vi "updateCamera.vi"(8 "error in (no error)":errorcluster, 10 "data":T1, 11 "AtomChipHWC in":refnum<class "AtomChipHWC.lvclass">) -> (0 "error out":errorcluster, 3 "AtomChipHWC out":refnum<class "AtomChipHWC.lvclass">)   [LabVIEW 2011, in "Hardware.lvlib" / "HWControllers.lvlib" / "AtomChipHWC.lvclass"]
uses:
  AtomChipHWC.lvclass
  AtomChipHWC.lvclass/AtomChipHWC.ctl
  Network Controllers/NetworkCamera/NetworkCamera.lvclass
panel:
  # "start - stop in type?"
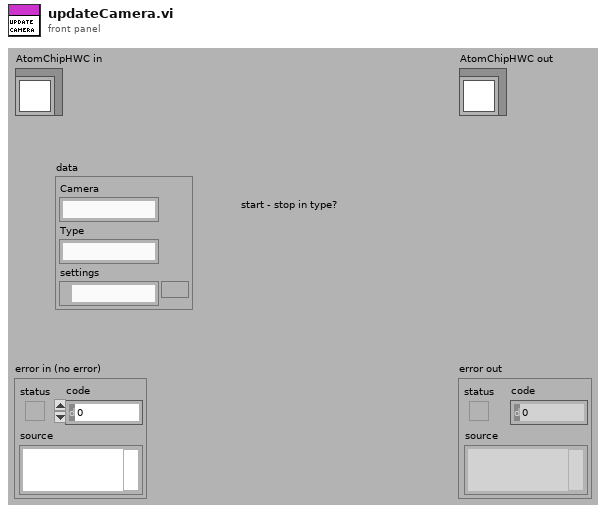
[diagram p1: front panel]
types:
  T1 = cluster{"Camera":string, "Type":string, "settings":path}
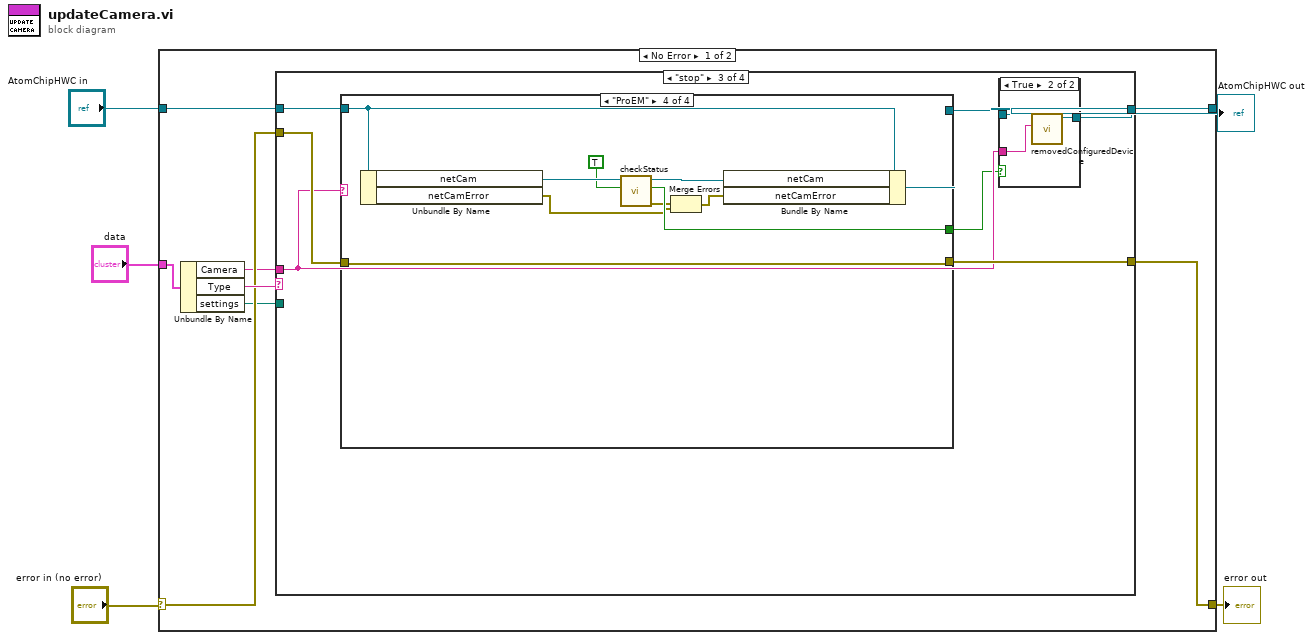
[diagram p0: block diagram]
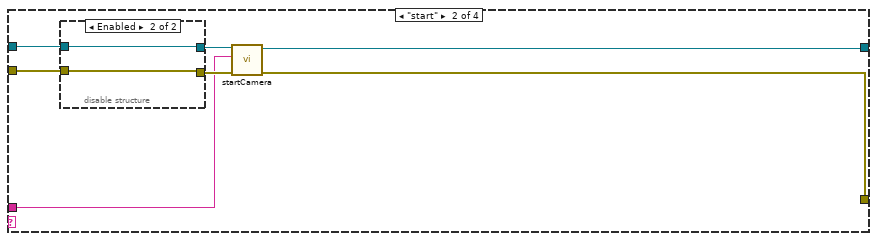
[diagram p3: hidden frame]
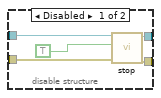
[diagram p4: hidden frame]
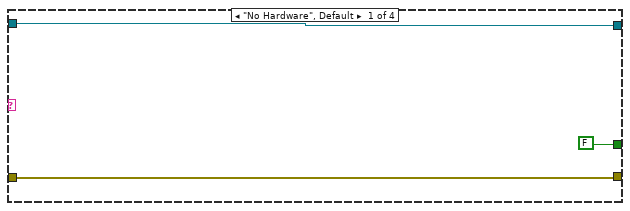
[diagram p6: hidden frame]
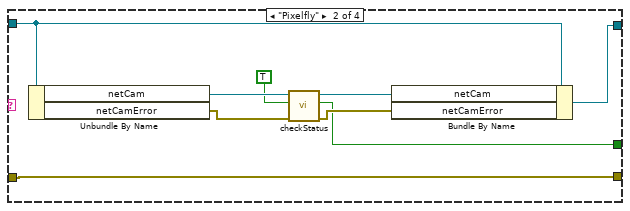
[diagram p7: hidden frame]
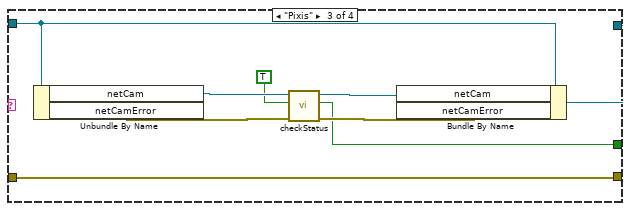
[diagram p8: hidden frame]
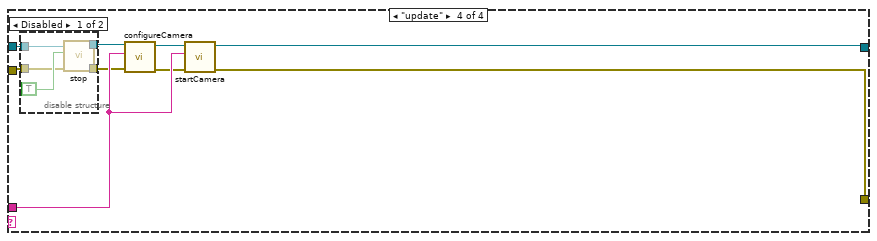
[diagram p9: hidden frame]
diagram:
  n1 = case shown="No Error" "error in (no error)" {
    selector: "error in (no error)" -> [w10 w88]
    tunnel: [w9 w89] -> w4
    tunnel: "AtomChipHWC in" -> [w11 w89]
    tunnel: [w8 w88] -> w2
    tunnel: "data" -> [w13 _]
    frame No Error {
      n2 = Unbundle By Name(w13) -> ("Camera"=w6:string, "Type"=w12:string, "settings"=w7:path)
      n3 = case shown="\"stop\"" w12 {
        tunnel: w11 -> [w15 w22 w36 w75]
        tunnel: w10 -> [w14 w21 w35 w72]
        tunnel: [w15 w18 w32 w77] -> w9
        tunnel: [w14 w17 w34 w76] -> w8
        tunnel: w7 -> [_ _ _ _]
        tunnel: w6 -> [_ w16 w31 w79]
        frame "", Default {
        }
        frame "start" {
          n4 = disable-structure shown="Enabled" {
            disable-tunnel: w22 -> [w26 w29]
            disable-tunnel: w21 -> [w25 w28]
            disable-tunnel: [w24 w29] -> w20
            disable-tunnel: [w23 w28] -> w19
            frame Disabled {
              n5 = call-dynamic "stop.vi"("error in (no error)"=w25, "stop?"=TRUE, "AtomChipHWC in"=w26) -> ("error out"=w23:errorcluster, "AtomChipHWC out"=w24:refnum<class "AtomChipHWC.lvclass">)  [unwired: 6 in, 1 out]
            }
            frame Enabled {
            }
          }
          n6 = call "startCamera.vi"("error in (no error)"=w19, "camera"=w16, "AtomChipHWC in"=w20) -> ("error out"=w17:errorcluster, "AtomChipHWC out"=w18:refnum<class "AtomChipHWC.lvclass">)  [unwired: 7 in]
        }
        frame "stop" {
          n7 = case shown="\"ProEM\"" w31 {
            tunnel: [w43 w51 w60 w70] -> w33
            tunnel: [w41 w44 w53 w65] -> w34
            tunnel: w36 -> [w43 w52 w61 w71]
            tunnel: [FALSE w45 w54 w66] -> w30
            tunnel: w35 -> [w41 w44 w53 w65]
            frame "No Hardware", Default {
            }
            frame "Pixelfly" {
              n8 = Unbundle By Name(w52) -> ("netCam"=w49:refnum<class "NetworkCamera.lvclass">, "netCamError"=w48:errorcluster)
              n9 = call-dynamic "checkStatus.vi"("error in (no error)"=w48, "stop"=TRUE, "NetworkCamera in"=w49) -> ("error out"=w47:errorcluster, "stopped?"=w45:bool, "NetworkCamera out"=w50:refnum<class "NetworkCamera.lvclass">)  [unwired: 6 in]
              n10 = Bundle By Name(cluster=w52, "netCam"=w50, "netCamError"=w47) -> (w51:refnum<class "AtomChipHWC.lvclass">)
            }
            frame "Pixis" {
              n11 = Unbundle By Name(w61) -> ("netCam"=w58:refnum<class "NetworkCamera.lvclass">, "netCamError"=w57:errorcluster)
              n12 = call-dynamic "checkStatus.vi"("error in (no error)"=w57, "stop"=TRUE, "NetworkCamera in"=w58) -> ("error out"=w56:errorcluster, "stopped?"=w54:bool, "NetworkCamera out"=w59:refnum<class "NetworkCamera.lvclass">)  [unwired: 6 in]
              n13 = Bundle By Name(cluster=w61, "netCam"=w59, "netCamError"=w56) -> (w60:refnum<class "AtomChipHWC.lvclass">)
            }
            frame "ProEM" {
              n14 = Unbundle By Name(w71) -> ("netCam"=w68:refnum<class "NetworkCamera.lvclass">, "netCamError"=w63:errorcluster)
              n15 = call-dynamic "checkStatus.vi"("stop"=TRUE, "NetworkCamera in"=w68) -> ("error out"=w64:errorcluster, "stopped?"=w66:bool, "NetworkCamera out"=w69:refnum<class "NetworkCamera.lvclass">)  [unwired: 7 in]
              n16 = Merge Errors(w64, w63) -> (w62:errorcluster)
              n17 = Bundle By Name(cluster=w71, "netCam"=w69, "netCamError"=w62) -> (w70:refnum<class "AtomChipHWC.lvclass">)
            }
          }
          n18 = case shown="True" w30 {
            tunnel: w33 -> [w37 w40]
            tunnel: [w37 w39] -> w32
            tunnel: w31 -> [_ w38]
            frame False {
            }
            frame True {
              n19 = call-dynamic "removedConfiguredDevice.vi"("device"=w38, "HWController in"=w40) -> ("HWController out"=w39:refnum<class "AtomChipHWC.lvclass">)  [unwired: 8 in, 1 out]
            }
          }
        }
        frame "update" {
          n20 = disable-structure shown="Disabled" {
            disable-tunnel: w75 -> [w84 w87]
            disable-tunnel: [w83 w87] -> w74
            disable-tunnel: [w82 w86] -> w73
            disable-tunnel: w72 -> [w81 w86]
            frame Disabled {
              n21 = call-dynamic "stop.vi"("error in (no error)"=w81, "stop?"=TRUE, "AtomChipHWC in"=w84) -> ("error out"=w82:errorcluster, "AtomChipHWC out"=w83:refnum<class "AtomChipHWC.lvclass">)  [unwired: 6 in, 1 out]
            }
            frame Enabled {
            }
          }
          n22 = call "configureCamera.vi"("error in (no error)"=w73, "device"=w79, "AtomChipHWC in"=w74) -> ("error out"=w78:errorcluster, "AtomChipHWC out"=w80:refnum<class "AtomChipHWC.lvclass">)  [unwired: 7 in]
          n23 = call "startCamera.vi"("error in (no error)"=w78, "camera"=w79, "AtomChipHWC in"=w80) -> ("error out"=w76:errorcluster, "AtomChipHWC out"=w77:refnum<class "AtomChipHWC.lvclass">)  [unwired: 7 in]
        }
      }
    }
    frame Error {
    }
  }
  "error out" <- w2
  "AtomChipHWC out" <- w4
